vi "CMD_WAIT.vi"(6 "Gantry in":refnum<class "Gantry.lvclass">, 8 "error in (no error)":errorcluster, 10 "Arguments":string[](array[string]), 11 "gScript Interpreter in":refnum<class "gScript Interpreter.lvclass">) -> (0 "error out":errorcluster, 3 "gScript Interpreter out":refnum<class "gScript Interpreter.lvclass">, 4 "Gantry out":refnum<class "Gantry.lvclass">)   [LabVIEW 2023, in "gScript Interpreter.lvclass"]
uses:
  gScript Interpreter.lvclass
  Shared Components/Gantry Class/Gantry.lvclass
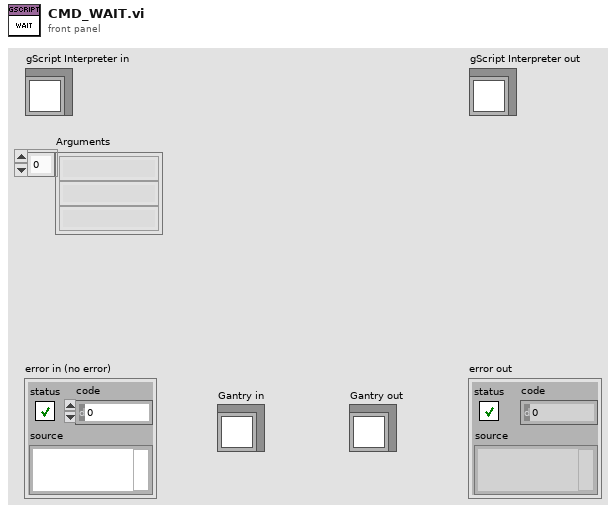
[diagram p1: front panel]
types:
  T1 = typedef "Memory Cell.ctl" = cluster{"type":T2, "x":dbl, "y":dbl, "z":dbl, "w":dbl}
  T2 = typedef "Memory Cell Type Enum.ctl" = enum16{"integer", "float", "vector", "rotation"}
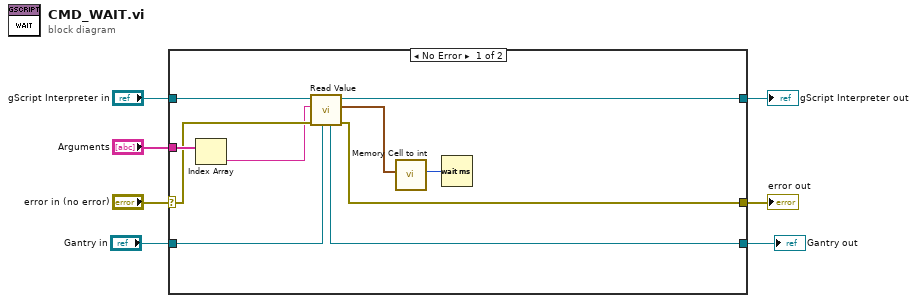
[diagram p0: block diagram]
diagram:
  n1 = case shown="No Error" "error in (no error)" {
    selector: "error in (no error)" -> [w15 w20]
    tunnel: [w12 w20] -> w6
    tunnel: [w11 w19] -> w4
    tunnel: "gScript Interpreter in" -> [w16 w19]
    tunnel: "Arguments" -> [w17 _]
    tunnel: "Gantry in" -> [w9 w18]
    tunnel: [w8 w18] -> w1
    frame No Error {
      n2 = Index Array(array=w17) -> (element=w10:string)  [unwired: 1 in]
      n3 = call-dynamic "Read Value.vi"("Gantry in"=w9, "error in (no error)"=w15, "String in"=w10, "gScript Interpreter in"=w16) -> ("error out"=w12:errorcluster, "Memory Cell"=w14:T1, "gScript Interpreter out"=w11:refnum<class "gScript Interpreter.lvclass">, "Gantry out"=w8:refnum<class "Gantry.lvclass">)  [unwired: 4 in]
      n4 = call "Memory Cell to int.vi"("Memory Cell"=w14) -> ("Int out"=w13:i32)  [unwired: 10 in]
      n5 = Wait (ms)(milliseconds to wait=w13) -> ()  [unwired: 1 out]
    }
    frame Error {
    }
  }
  "error out" <- w6
  "gScript Interpreter out" <- w4
  "Gantry out" <- w1
